vi "Begin.vi"(8 "error in (no error)":errorcluster, 10 "Configuration In":variant, 11 "Cargo in":refnum<class "Cargo.lvclass">) -> (0 "error out":errorcluster, 3 "Cargo out":refnum<class "Cargo.lvclass">)   [LabVIEW 2018, in "Cargo.lvlib" / "Cargo.lvclass"]
doc: "use this VI to open references to motors"
uses:
  Cargo.lvclass
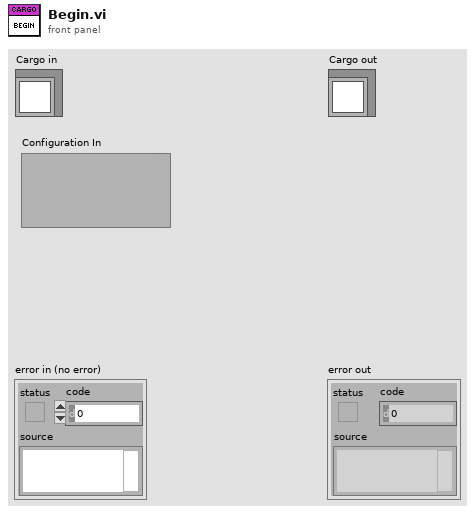
[diagram p1: front panel]
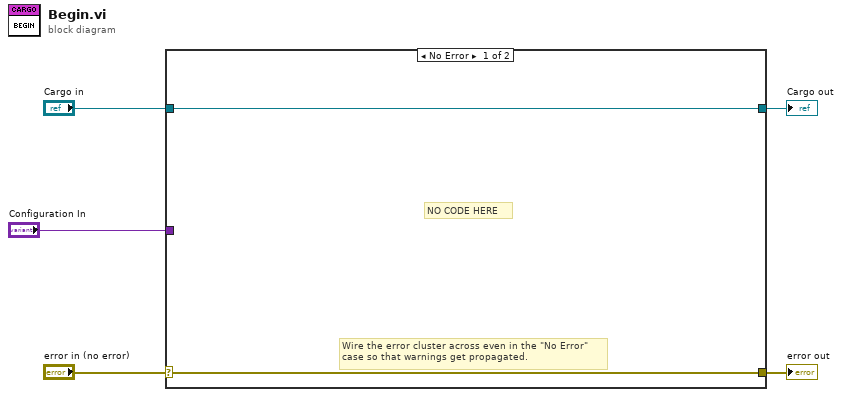
[diagram p0: block diagram]
diagram:
  n1 = case shown="No Error" "error in (no error)" {
    selector: "error in (no error)" -> [w6 w9]
    tunnel: [w6 w9] -> w4
    tunnel: [w7 w8] -> w2
    tunnel: "Cargo in" -> [w7 w8]
    tunnel: "Configuration In" -> [_ _]
    frame No Error {
      # "NO CODE HERE"
      # "Wire the error cluster across even in the \"No Error\"\ncase so that warnings get propagated."
    }
    frame Error {
    }
  }
  "error out" <- w4
  "Cargo out" <- w2
